vi "Autonomous Independent.vi"   [LabVIEW 2017]
doc: "This VI is called when autonomous begins, and will automatically be terminated when autonomous ends. You can carry out timed or sensor driven robot movement independently without needing to return to the caller."
uses:
  <vilib>/Rock Robotics/WPI/Utilities/WPI_GetSetVariantRefNum.vi
  <vilib>/Rock Robotics/Network Tables/NT Read String.vi
  <vilib>/Rock Robotics/Network Tables/NT Write Numeric Array.vi
  <vilib>/Rock Robotics/WPI/RobotDrive/WPI_RobotDriveArcadeDrive_Standard(NoSaturation).vi
panel:
  # "Be sure to right-click and choose Data Operations>>Make Current Value default if you want to save the array values with the VI"
types:
  T1 = typedef "WPI_JoystickDevRef.ctl" = cluster{"Device":T2}
  T2 = typedef "WPI_JoystickDeviceEnum.ctl" = enum16{"USB 0", "USB 1", "USB 2", "USB 3", "USB 4", "USB 5"}
  T3 = typedef "WPI_RobotDriveDevRef.ctl" = cluster{"DevStatus":errorcluster, "Motors[]":T4[], "Square Inputs":bool, "Max Output":dbl}
  T4 = typedef "WPI_MotorControlDeviceRef.ctl" = cluster{"DeviceStatus":errorcluster, "Type":T5, "PWM":cluster{"PWM Channel":T6, "DeadBand":T7}, "CAN":cluster{"Device Number":u8, "SetOutput VI Ref":variant, "GetOutput VI Ref":variant, "Enable VI Ref":variant, "Disable VI Ref":variant, "Data":variant}, "Invert":bool, "DIO PWM":cluster{"PWM \"Enable\" Channel":T6, "DIOChannel":T8, "PWM Rate":dbl}}
  T5 = typedef "WPI_MotorControlType.ctl" = enum16{"PWM", "CAN", "DIO PWM"}
  T6 = typedef "FPGA_DIOPWMChannel.ctl" = enum8{"PWM 0", "PWM 1", "PWM 2", "PWM 3", "PWM 4", "PWM 5", "PWM 6", "PWM 7", "PWM 8", "PWM 9", "PWM MXP 0", "PWM MXP 1", "PWM MXP 2", "PWM MXP 3", "PWM MXP 4", "PWM MXP 5", "PWM MXP 6", "PWM MXP 7", "PWM MXP 8", "PWM MXP 9", "Invalid"}
  T7 = typedef "WPI_PWMDeadband.ctl" = cluster{"Name":string, "maxPositivePwm":i32, "minPositivePwm":i32, "centerPwm":i32, "maxNegativePwm":i32, "minNegativePwm":i32, "angularRange":u16}
  T8 = typedef "FPGA_DIOChannel.ctl" = enum8{"DIO 0", "DIO 1", "DIO 2", "DIO 3", "DIO 4", "DIO 5", "DIO 6", "DIO 7", "DIO 8", "DIO 9", "DIO MXP 0", "DIO MXP 1", "DIO MXP 2", "DIO MXP 3", "DIO MXP 4", "DIO MXP 5", "DIO MXP 6", "DIO MXP 7", "DIO MXP 8", "DIO MXP 9", "DIO MXP 10", "DIO MXP 11", "DIO MXP 12", "DIO MXP 13", "DIO MXP 14", "DIO MXP 15", "SPI Port CS1", "SPI Port CS2", "SPI Port CS3", "SPI Port MISO", "SPI Port MOSI", "Invalid"}
  T9 = typedef "WPI_SwitchDevRef.ctl" = cluster{"DevStatus":errorcluster, "DIO Channel":T8, "CntIndex":T10, "Normally Closed":bool}
  T10 = typedef "FPGA_CounterCtrSystemIndex.ctl" = enum8{"Ctr 0", "Ctr 1", "Ctr 2", "Ctr 3", "Ctr 4", "Ctr 5", "Ctr 6", "Ctr 7", "Invalid"}
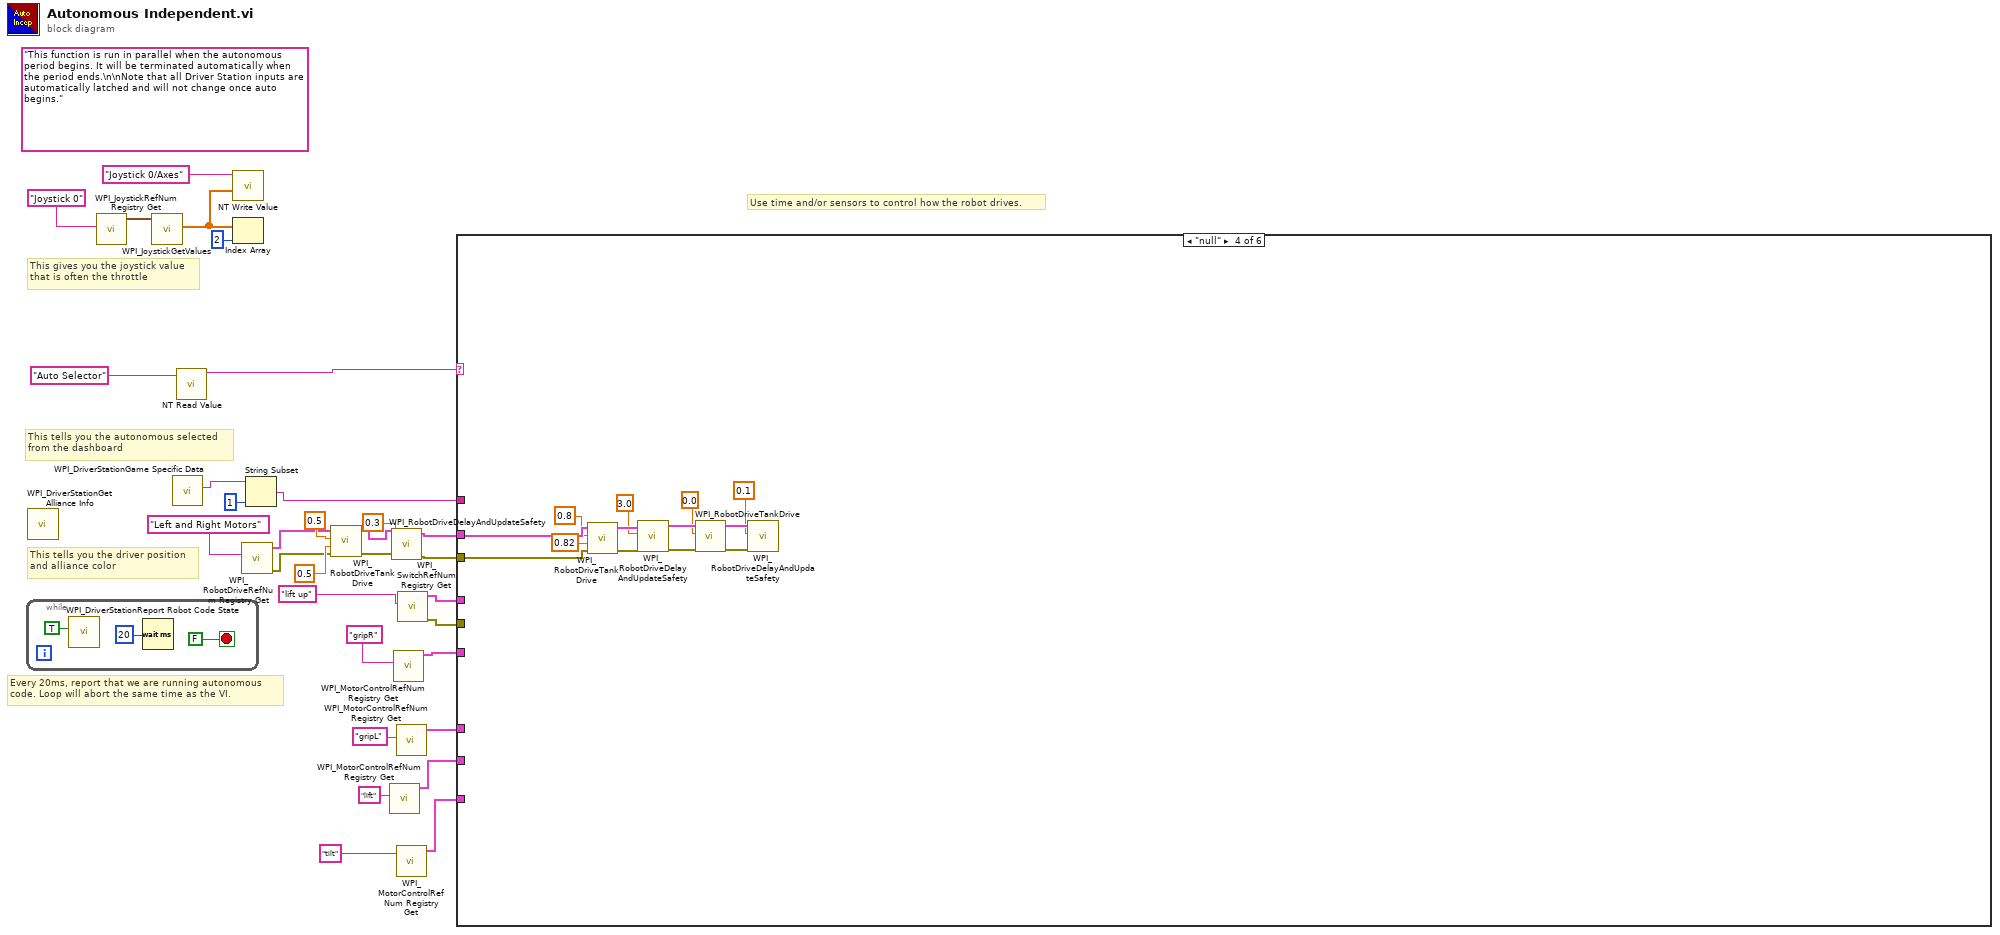
[diagram p0: block diagram]
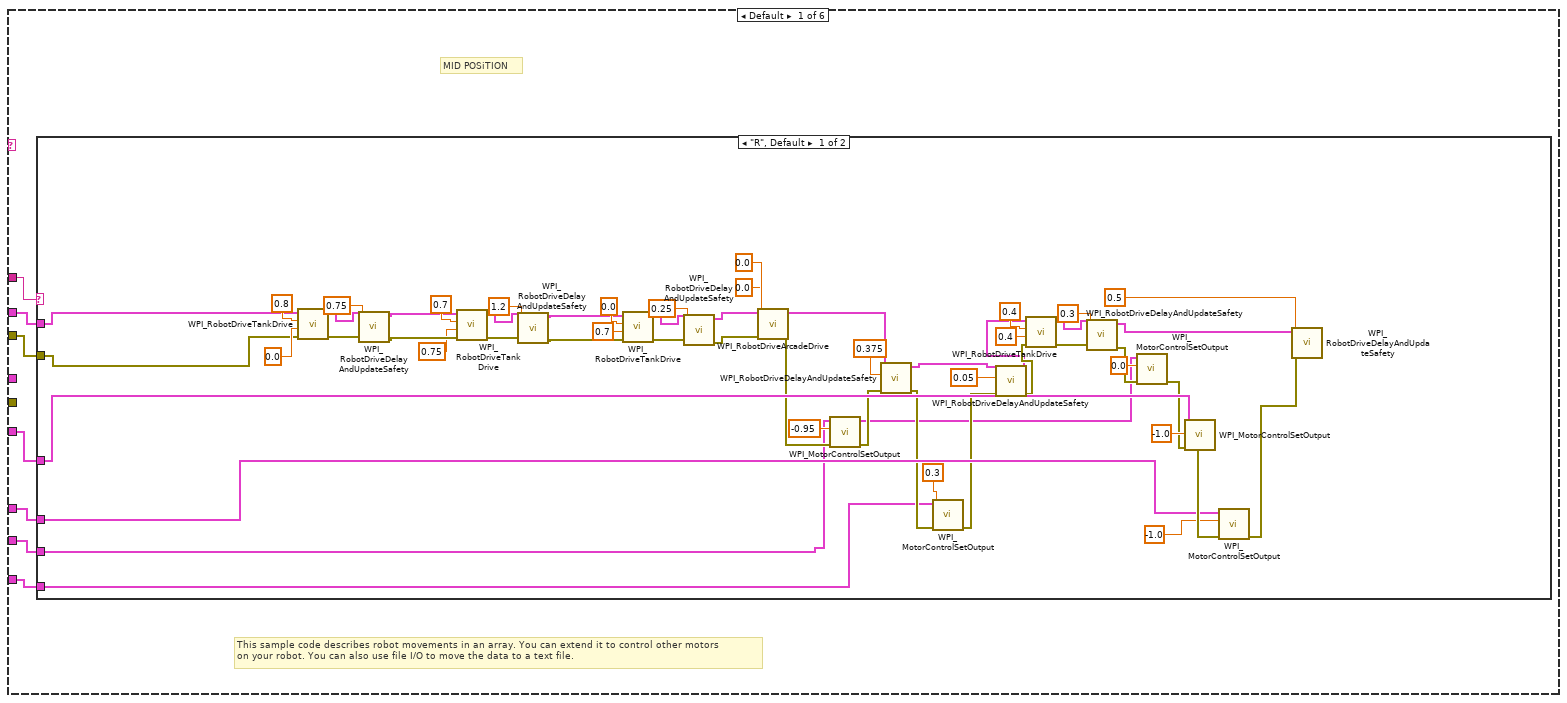
[diagram p2: hidden frame]
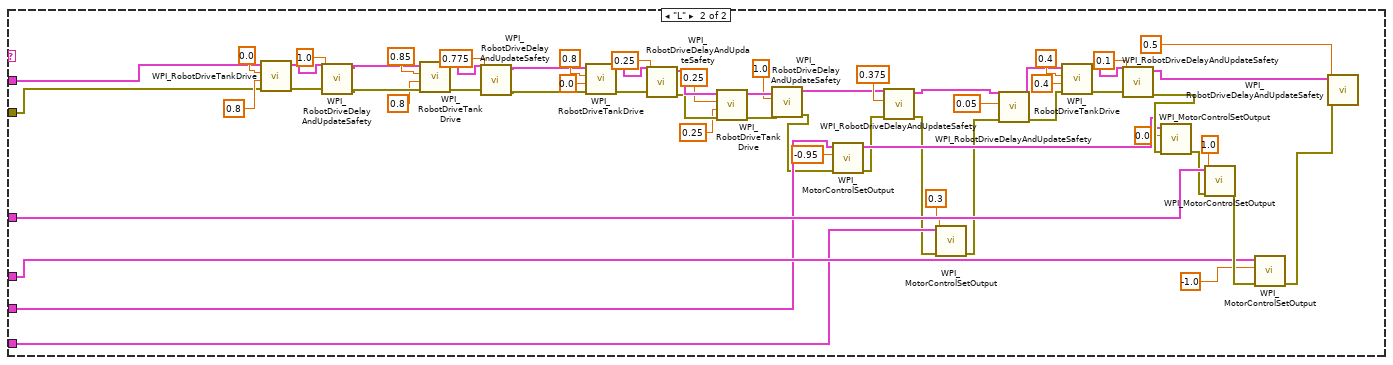
[diagram p3: hidden frame]
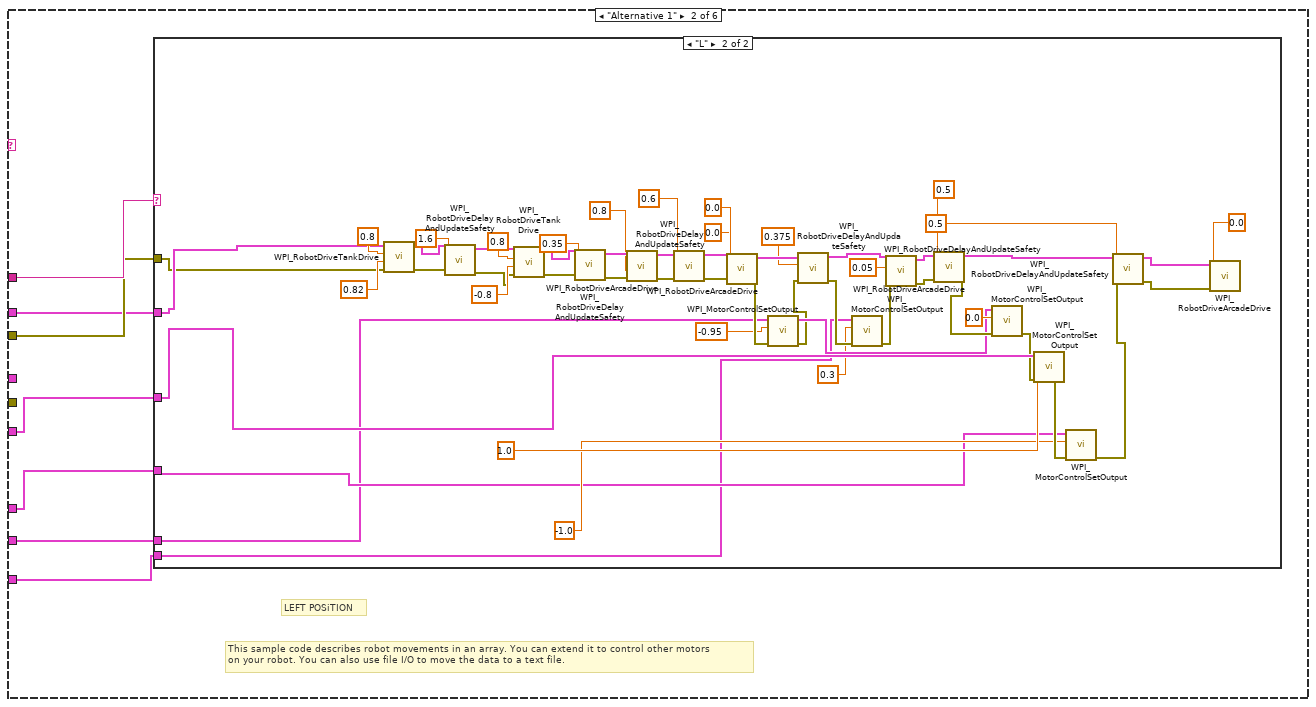
[diagram p4: hidden frame]
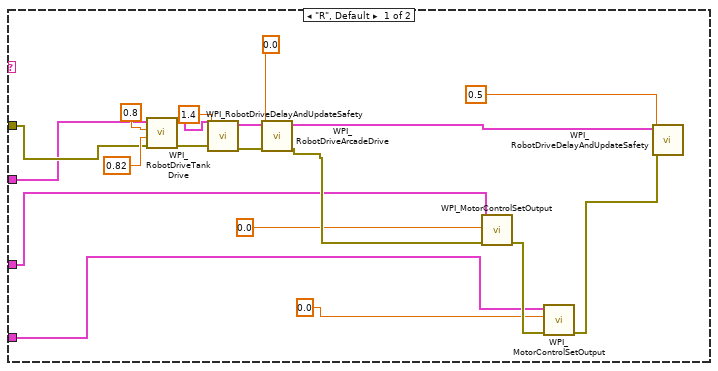
[diagram p5: hidden frame]
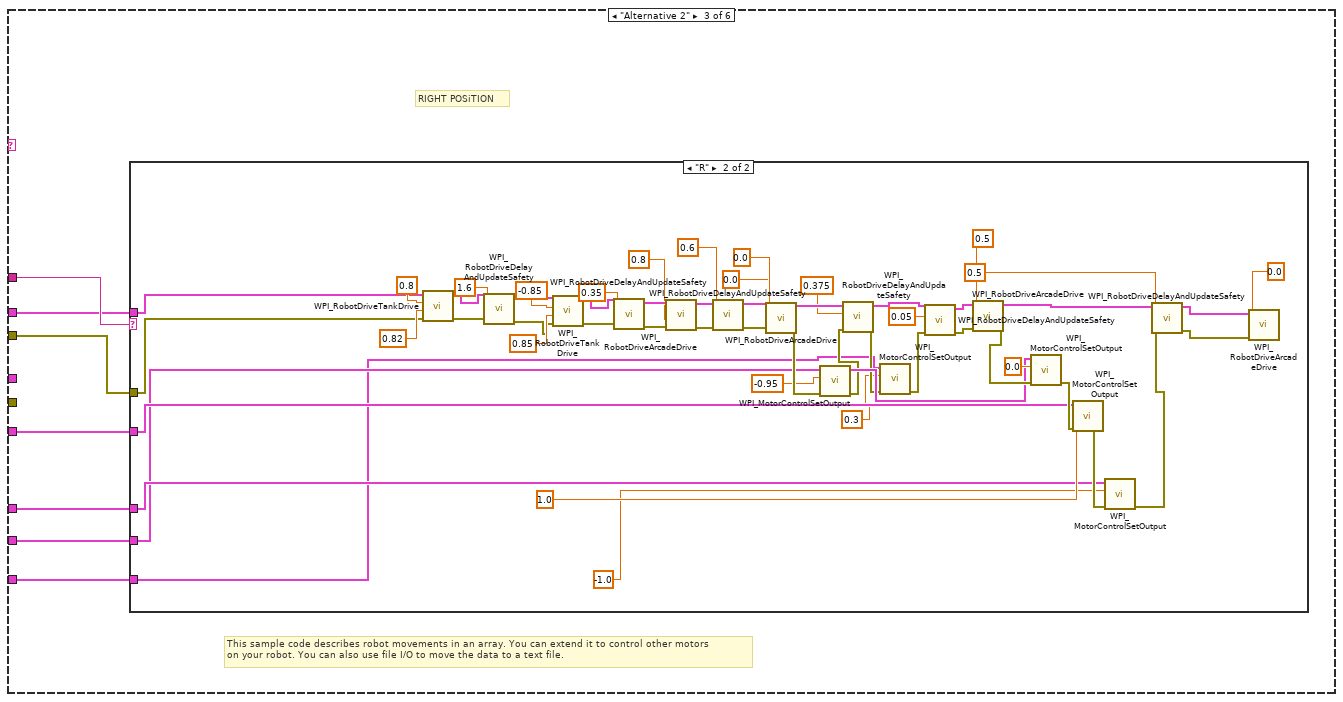
[diagram p6: hidden frame]
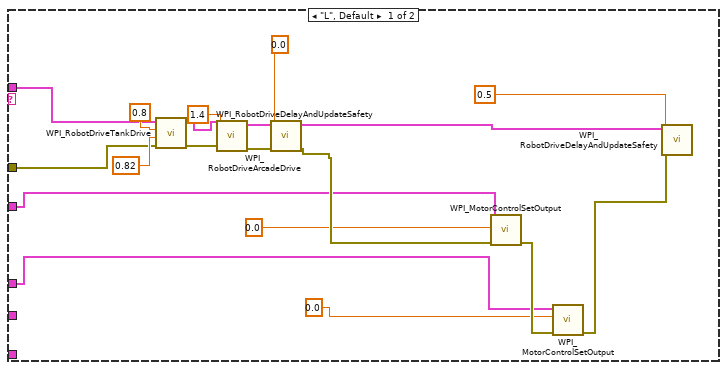
[diagram p7: hidden frame]
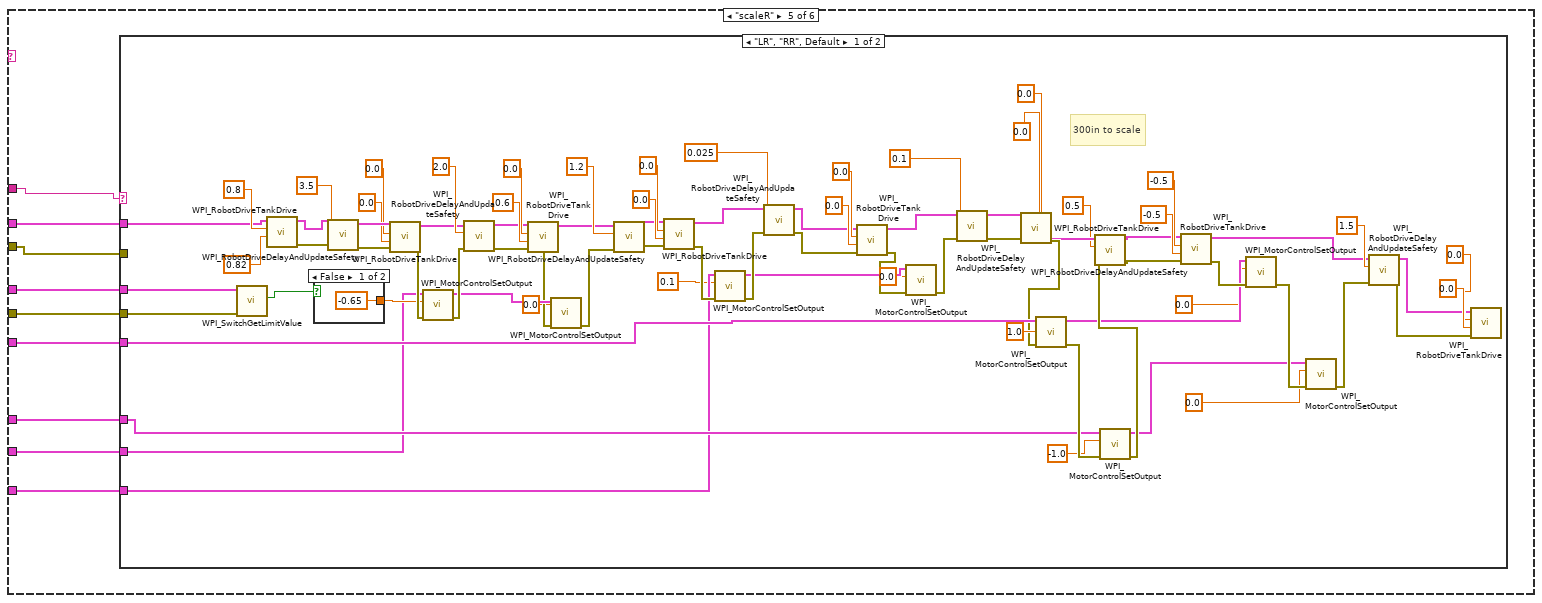
[diagram p8: hidden frame]
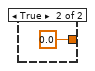
[diagram p9: hidden frame]
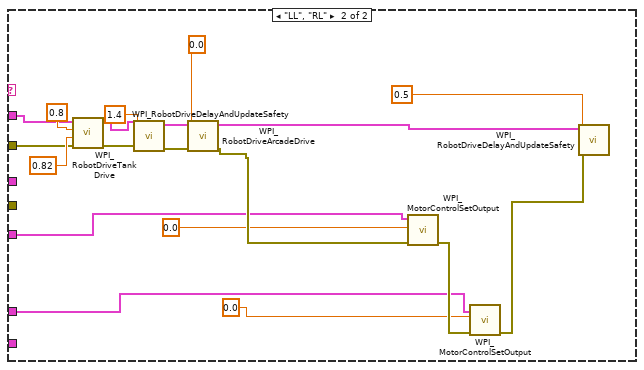
[diagram p10: hidden frame]
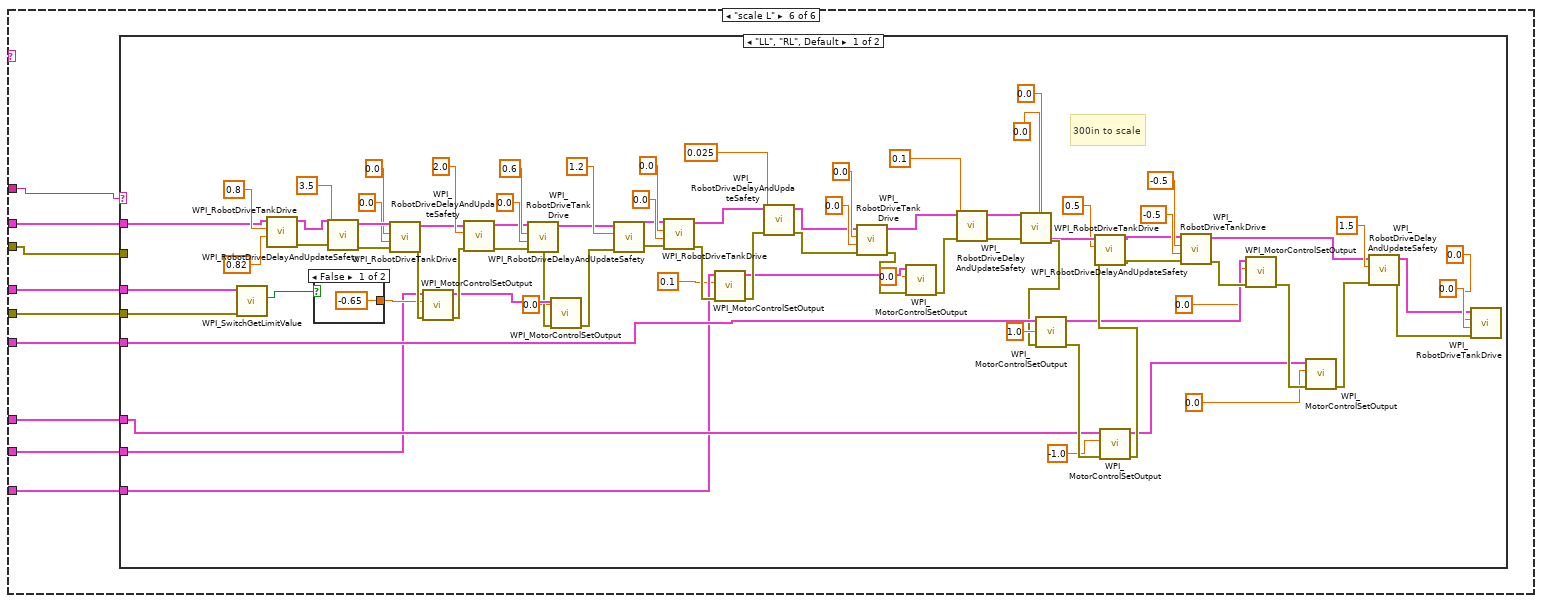
[diagram p11: hidden frame]
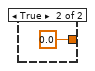
[diagram p12: hidden frame]
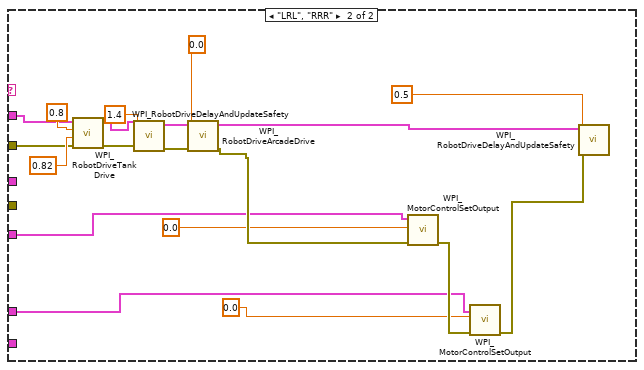
[diagram p13: hidden frame]
diagram:
  (unwired) "This function is run in parallel when the autonomous period begins. It will be terminated automatically when the period ends.\n\nNote that all Driver Station inputs are automatically latched and will not change once auto begins."
  # "This tells you the autonomous selected\nfrom the dashboard"
  # "Every 20ms, report that we are running autonomous\ncode. Loop will abort the same time as the VI."
  # "This gives you the joystick value\nthat is often the throttle"
  # "Use time and/or sensors to control how the robot drives."
  # "This tells you the driver position\nand alliance color"
  n1 = while {
    stop <- FALSE stop-if-true
    n2 = call <vilib>:"WPI_DriverStationReport Robot Code State.vi"("Autonomous"=TRUE) -> ()  [unwired: 10 in, 1 out]
    n3 = Wait (ms)(milliseconds to wait=u32 20) -> ()  [unwired: 1 out]
  }
  n4 = call <vilib>:"WPI_DriverStationGet Alliance Info.vi"() -> ()  [unwired: 12 out]
  n5 = call <vilib>:"WPI_JoystickRefNum Registry Get.vi"("refnum name"="Joystick 0") -> ("JoystickDevRef"=w30:T1)  [unwired: 1 in, 9 out]
  n6 = call <vilib>:"WPI_JoystickGetValues.vi"("JoystickDevRef"=w30) -> ("Axes"=w26:dbl[])  [unwired: 6 in, 4 out]
  n7 = call <vilib>:"WPI_DriverStationGame Specific Data.vi"() -> ("Game Specific Data"=w24:string)  [unwired: 11 in]
  n8 = call-poly <vilib>:"NT Read Value.vi"("Name"="Auto Selector") -> ("String"=w27:string)  [unwired: 9 in, 1 out]
  n9 = call-poly <vilib>:"NT Write Value.vi"("Numeric Array"=w26, "Name"="Joystick 0/Axes") -> ()  [unwired: 9 in, 1 out]
  n10 = Index Array(array=w26, index=2) -> ()  [unwired: 1 out]
  n11 = call <vilib>:"WPI_RobotDriveRefNum Registry Get.vi"("refnum name"="Left and Right Motors") -> ("error out"=w6:errorcluster, "RobotDriveDevRef"=w5:T3)  [unwired: 1 in, 8 out]
  n12 = String Subset(string=w24, length (rest)=1 ("length (rest)")) -> (substring=w22:string)  [unwired: 1 in]
  n13 = call <vilib>:"WPI_RobotDriveTankDrive.vi"("error in (no error)"=w6, "Right axis value"=0.5 ("Y axis value"), "Left axis value"=0.5 ("X axis value"), "RobotDriveDevRef"=w5) -> ("error out"=w10:errorcluster, "RobotDriveDevRef"=w9:T3)  [unwired: 5 in, 1 out]
  n14 = call <vilib>:"WPI_MotorControlRefNum Registry Get.vi"("refnum name"="lift") -> ("MotorControlDevRef"=w12:T4)  [unwired: 9 in, 1 out]
  n15 = call <vilib>:"WPI_RobotDriveDelayAndUpdateSafety.vi"("error in (no error)"=w10, "Delay (s)"=0.3, "RobotDriveDevRef"=w9) -> ("error out"=w3:errorcluster, "RobotDriveDevRef 2"=w4:T3)  [unwired: 7 in]
  n16 = call <vilib>:"WPI_MotorControlRefNum Registry Get.vi"("refnum name"="gripR") -> ("MotorControlDevRef"=w19:T4)  [unwired: 9 in, 1 out]
  n17 = call <vilib>:"WPI_MotorControlRefNum Registry Get.vi"("refnum name"="gripL") -> ("MotorControlDevRef"=w17:T4)  [unwired: 9 in, 1 out]
  n18 = call <vilib>:"WPI_MotorControlRefNum Registry Get.vi"("refnum name"="tilt") -> ("MotorControlDevRef"=w2:T4)  [unwired: 9 in, 1 out]
  n19 = call <vilib>:"WPI_SwitchRefNum Registry Get.vi"("refnum name"="lift up") -> ("error out"=w14:errorcluster, "SwitchDevRef"=w13:T9)  [unwired: 9 in]
  n20 = case shown="\"null\"" w27 {
    tunnel: w22 -> [w41 w163 w243 _ w338 w447]
    tunnel: w3 -> [w40 w162 w242 w326 w331 w440]
    tunnel: w19 -> [w39 w161 w241 _ w335 w444]
    tunnel: w17 -> [w38 w160 w240 _ w336 w445]
    tunnel: w4 -> [w37 w159 w239 w327 w337 w446]
    tunnel: w14 -> [_ _ _ _ w334 w443]
    tunnel: w13 -> [_ _ _ _ w333 w442]
    tunnel: w12 -> [w36 w158 w238 _ w332 w441]
    tunnel: w2 -> [w35 w157 w237 _ w330 w439]
    frame Default {
      # "MID POSiTION"
      # "This sample code describes robot movements in an array. You can extend it to control other motors\non your robot. You can also use file I/O to move the data to a text file."
      n21 = case shown="\"R\", Default" w41 {
        tunnel: w40 -> [w87 w126]
        tunnel: w39 -> [w86 w125]
        tunnel: w38 -> [w85 w124]
        tunnel: w37 -> [w64 w123]
        tunnel: w36 -> [w47 w116]
        tunnel: w35 -> [w46 w111]
        frame "R", Default {
          n22 = call <vilib>:"WPI_RobotDriveTankDrive.vi"("error in (no error)"=w87, "Right axis value"=0.0 ("Y axis value"), "Left axis value"=0.8 ("X axis value"), "RobotDriveDevRef"=w64) -> ("error out"=w93:errorcluster, "RobotDriveDevRef"=w92:T3)  [unwired: 5 in, 1 out]
          n23 = call <vilib>:"WPI_RobotDriveDelayAndUpdateSafety.vi"("error in (no error)"=w93, "Delay (s)"=0.75, "RobotDriveDevRef"=w92) -> ("error out"=w79:errorcluster, "RobotDriveDevRef 2"=w80:T3)  [unwired: 7 in]
          n24 = call <vilib>:"WPI_RobotDriveTankDrive.vi"("error in (no error)"=w79, "Right axis value"=0.75, "Left axis value"=0.7 ("X axis value"), "RobotDriveDevRef"=w80) -> ("error out"=w83:errorcluster, "RobotDriveDevRef"=w82:T3)  [unwired: 5 in, 1 out]
          n25 = call <vilib>:"WPI_RobotDriveDelayAndUpdateSafety.vi"("error in (no error)"=w83, "Delay (s)"=1.2, "RobotDriveDevRef"=w82) -> ("error out"=w72:errorcluster, "RobotDriveDevRef 2"=w73:T3)  [unwired: 7 in]
          n26 = call <vilib>:"WPI_RobotDriveTankDrive.vi"("error in (no error)"=w72, "Right axis value"=0.7, "Left axis value"=0.0 ("X axis value"), "RobotDriveDevRef"=w73) -> ("error out"=w76:errorcluster, "RobotDriveDevRef"=w75:T3)  [unwired: 5 in, 1 out]
          n27 = call <vilib>:"WPI_RobotDriveDelayAndUpdateSafety.vi"("error in (no error)"=w76, "Delay (s)"=0.25, "RobotDriveDevRef"=w75) -> ("error out"=w60:errorcluster, "RobotDriveDevRef 2"=w61:T3)  [unwired: 7 in]
          n28 = call-poly <vilib>:"WPI_RobotDriveArcadeDrive.vi"("error in (no error)"=w60, "Y axis value"=0.0, "X axis value"=0.0, "RobotDriveDevRef"=w61) -> ("error out"=w52:errorcluster, "RobotDriveDevRef"=w53:T3)  [unwired: 5 in, 1 out]
          n29 = call <vilib>:"WPI_MotorControlSetOutput.vi"("error in (no error)"=w52, "Output"=-0.95, "MotorControlDevRef"=w47) -> ("error out"=w51:errorcluster, "MotorControlDevRef"=w45:T4)  [unwired: 6 in, 1 out]
          n30 = call <vilib>:"WPI_RobotDriveDelayAndUpdateSafety.vi"("error in (no error)"=w51, "Delay (s)"=0.375 ("Output"), "RobotDriveDevRef"=w53) -> ("error out"=w50:errorcluster, "RobotDriveDevRef 2"=w44:T3)  [unwired: 7 in]
          n31 = call <vilib>:"WPI_MotorControlSetOutput.vi"("error in (no error)"=w50, "Output"=0.3, "MotorControlDevRef"=w46) -> ("error out"=w49:errorcluster)  [unwired: 6 in, 2 out]
          n32 = call <vilib>:"WPI_RobotDriveDelayAndUpdateSafety.vi"("error in (no error)"=w49, "Delay (s)"=0.05, "RobotDriveDevRef"=w44) -> ("error out"=w48:errorcluster, "RobotDriveDevRef 2"=w43:T3)  [unwired: 7 in]
          n33 = call <vilib>:"WPI_RobotDriveTankDrive.vi"("error in (no error)"=w48, "Right axis value"=0.4, "Left axis value"=0.4 ("X axis value"), "RobotDriveDevRef"=w43) -> ("error out"=w69:errorcluster, "RobotDriveDevRef"=w68:T3)  [unwired: 5 in, 1 out]
          n34 = call <vilib>:"WPI_RobotDriveDelayAndUpdateSafety.vi"("error in (no error)"=w69, "Delay (s)"=0.3, "RobotDriveDevRef"=w68) -> ("error out"=w59:errorcluster, "RobotDriveDevRef 2"=w65:T3)  [unwired: 7 in]
          n35 = call <vilib>:"WPI_MotorControlSetOutput.vi"("error in (no error)"=w59, "Output"=0.0, "MotorControlDevRef"=w45) -> ("error out"=w57:errorcluster)  [unwired: 6 in, 2 out]
          n36 = call <vilib>:"WPI_MotorControlSetOutput.vi"("error in (no error)"=w57, "Output"=-1.0, "MotorControlDevRef"=w86) -> ("error out"=w95:errorcluster)  [unwired: 6 in, 2 out]
          n37 = call <vilib>:"WPI_MotorControlSetOutput.vi"("error in (no error)"=w95, "Output"=-1.0, "MotorControlDevRef"=w85) -> ("error out"=w94:errorcluster)  [unwired: 6 in, 2 out]
          n38 = call <vilib>:"WPI_RobotDriveDelayAndUpdateSafety.vi"("error in (no error)"=w94, "Delay (s)"=0.5, "RobotDriveDevRef"=w65) -> ()  [unwired: 7 in, 2 out]
        }
        frame "L" {
          n39 = call <vilib>:"WPI_RobotDriveTankDrive.vi"("error in (no error)"=w126, "Right axis value"=0.8 ("Y axis value"), "Left axis value"=0.0 ("X axis value"), "RobotDriveDevRef"=w123) -> ("error out"=w152:errorcluster, "RobotDriveDevRef"=w151:T3)  [unwired: 5 in, 1 out]
          n40 = call <vilib>:"WPI_RobotDriveDelayAndUpdateSafety.vi"("error in (no error)"=w152, "Delay (s)"=1.0, "RobotDriveDevRef"=w151) -> ("error out"=w141:errorcluster, "RobotDriveDevRef 2"=w142:T3)  [unwired: 7 in]
          n41 = call <vilib>:"WPI_RobotDriveTankDrive.vi"("error in (no error)"=w141, "Right axis value"=0.8, "Left axis value"=0.85 ("X axis value"), "RobotDriveDevRef"=w142) -> ("error out"=w145:errorcluster, "RobotDriveDevRef"=w144:T3)  [unwired: 5 in, 1 out]
          n42 = call <vilib>:"WPI_RobotDriveDelayAndUpdateSafety.vi"("error in (no error)"=w145, "Delay (s)"=0.775, "RobotDriveDevRef"=w144) -> ("error out"=w134:errorcluster, "RobotDriveDevRef 2"=w135:T3)  [unwired: 7 in]
          n43 = call <vilib>:"WPI_RobotDriveTankDrive.vi"("error in (no error)"=w134, "Right axis value"=0.0, "Left axis value"=0.8 ("X axis value"), "RobotDriveDevRef"=w135) -> ("error out"=w138:errorcluster, "RobotDriveDevRef"=w137:T3)  [unwired: 5 in, 1 out]
          n44 = call <vilib>:"WPI_RobotDriveDelayAndUpdateSafety.vi"("error in (no error)"=w138, "Delay (s)"=0.25, "RobotDriveDevRef"=w137) -> ("error out"=w119:errorcluster, "RobotDriveDevRef 2"=w120:T3)  [unwired: 7 in]
          n45 = call <vilib>:"WPI_RobotDriveTankDrive.vi"("error in (no error)"=w119, "Right axis value"=0.25 ("X axis value"), "Left axis value"=0.25 ("X axis value"), "RobotDriveDevRef"=w120) -> ("error out"=w102:errorcluster, "RobotDriveDevRef"=w104:T3)  [unwired: 5 in, 1 out]
          n46 = call <vilib>:"WPI_RobotDriveDelayAndUpdateSafety.vi"("error in (no error)"=w102, "Delay (s)"=1.0 ("X axis value"), "RobotDriveDevRef"=w104) -> ("error out"=w101:errorcluster, "RobotDriveDevRef 2"=w103:T3)  [unwired: 7 in]
          n47 = call <vilib>:"WPI_MotorControlSetOutput.vi"("error in (no error)"=w101, "Output"=-0.95, "MotorControlDevRef"=w116) -> ("error out"=w109:errorcluster, "MotorControlDevRef"=w113:T4)  [unwired: 6 in, 1 out]
          n48 = call <vilib>:"WPI_RobotDriveDelayAndUpdateSafety.vi"("error in (no error)"=w109, "Delay (s)"=0.375 ("Output"), "RobotDriveDevRef"=w103) -> ("error out"=w108:errorcluster, "RobotDriveDevRef 2"=w105:T3)  [unwired: 7 in]
          n49 = call <vilib>:"WPI_MotorControlSetOutput.vi"("error in (no error)"=w108, "Output"=0.3, "MotorControlDevRef"=w111) -> ("error out"=w107:errorcluster)  [unwired: 6 in, 2 out]
          n50 = call <vilib>:"WPI_RobotDriveDelayAndUpdateSafety.vi"("error in (no error)"=w107, "Delay (s)"=0.05, "RobotDriveDevRef"=w105) -> ("error out"=w117:errorcluster, "RobotDriveDevRef 2"=w118:T3)  [unwired: 7 in]
          n51 = call <vilib>:"WPI_RobotDriveTankDrive.vi"("error in (no error)"=w117, "Right axis value"=0.4, "Left axis value"=0.4 ("X axis value"), "RobotDriveDevRef"=w118) -> ("error out"=w131:errorcluster, "RobotDriveDevRef"=w130:T3)  [unwired: 5 in, 1 out]
          n52 = call <vilib>:"WPI_RobotDriveDelayAndUpdateSafety.vi"("error in (no error)"=w131, "Delay (s)"=0.1, "RobotDriveDevRef"=w130) -> ("error out"=w115:errorcluster, "RobotDriveDevRef 2"=w127:T3)  [unwired: 7 in]
          n53 = call <vilib>:"WPI_MotorControlSetOutput.vi"("error in (no error)"=w115, "Output"=0.0, "MotorControlDevRef"=w113) -> ("error out"=w114:errorcluster)  [unwired: 6 in, 2 out]
          n54 = call <vilib>:"WPI_MotorControlSetOutput.vi"("error in (no error)"=w114, "Output"=1.0, "MotorControlDevRef"=w125) -> ("error out"=w154:errorcluster)  [unwired: 6 in, 2 out]
          n55 = call <vilib>:"WPI_MotorControlSetOutput.vi"("error in (no error)"=w154, "Output"=-1.0, "MotorControlDevRef"=w124) -> ("error out"=w153:errorcluster)  [unwired: 6 in, 2 out]
          n56 = call <vilib>:"WPI_RobotDriveDelayAndUpdateSafety.vi"("error in (no error)"=w153, "Delay (s)"=0.5, "RobotDriveDevRef"=w127) -> ()  [unwired: 7 in, 2 out]
        }
      }
    }
    frame "Alternative 1" {
      # "LEFT POSiTION"
      # "This sample code describes robot movements in an array. You can extend it to control other motors\non your robot. You can also use file I/O to move the data to a text file."
      n57 = case shown="\"L\"" w163 {
        tunnel: w162 -> [w167 w216]
        tunnel: w161 -> [w166 w215]
        tunnel: w160 -> [w165 w214]
        tunnel: w159 -> [w164 w217]
        tunnel: w158 -> [_ w194]
        tunnel: w157 -> [_ w184]
        frame "R", Default {
          n58 = call <vilib>:"WPI_RobotDriveTankDrive.vi"("error in (no error)"=w167, "Right axis value"=0.82 ("Y axis value"), "Left axis value"=0.8 ("X axis value"), "RobotDriveDevRef"=w164) -> ("error out"=w173:errorcluster, "RobotDriveDevRef"=w172:T3)  [unwired: 5 in, 1 out]
          n59 = call <vilib>:"WPI_RobotDriveDelayAndUpdateSafety.vi"("error in (no error)"=w173, "Delay (s)"=1.4, "RobotDriveDevRef"=w172) -> ("error out"=w181:errorcluster, "RobotDriveDevRef 2"=w180:T3)  [unwired: 7 in]
          n60 = call-poly <vilib>:"WPI_RobotDriveArcadeDrive.vi"("error in (no error)"=w181, "Y axis value"=0.0, "RobotDriveDevRef"=w180) -> ("error out"=w175:errorcluster, "RobotDriveDevRef"=w178:T3)  [unwired: 6 in, 1 out]
          n61 = call <vilib>:"WPI_MotorControlSetOutput.vi"("error in (no error)"=w175, "Output"=0.0, "MotorControlDevRef"=w166) -> ("error out"=w176:errorcluster)  [unwired: 6 in, 2 out]
          n62 = call <vilib>:"WPI_MotorControlSetOutput.vi"("error in (no error)"=w176, "Output"=0.0, "MotorControlDevRef"=w165) -> ("error out"=w174:errorcluster)  [unwired: 6 in, 2 out]
          n63 = call <vilib>:"WPI_RobotDriveDelayAndUpdateSafety.vi"("error in (no error)"=w174, "Delay (s)"=0.5, "RobotDriveDevRef"=w178) -> ()  [unwired: 7 in, 2 out]
        }
        frame "L" {
          n64 = call <vilib>:"WPI_RobotDriveTankDrive.vi"("error in (no error)"=w216, "Right axis value"=0.82 ("Y axis value"), "Left axis value"=0.8 ("X axis value"), "RobotDriveDevRef"=w217) -> ("error out"=w230:errorcluster, "RobotDriveDevRef"=w229:T3)  [unwired: 5 in, 1 out]
          n65 = call <vilib>:"WPI_RobotDriveDelayAndUpdateSafety.vi"("error in (no error)"=w230, "Delay (s)"=1.6, "RobotDriveDevRef"=w229) -> ("error out"=w218:errorcluster, "RobotDriveDevRef 2"=w219:T3)  [unwired: 7 in]
          n66 = call <vilib>:"WPI_RobotDriveTankDrive.vi"("error in (no error)"=w218, "Right axis value"=-0.8 ("Y axis value"), "Left axis value"=0.8 ("X axis value"), "RobotDriveDevRef"=w219) -> ("error out"=w223:errorcluster, "RobotDriveDevRef"=w222:T3)  [unwired: 5 in, 1 out]
          n67 = call <vilib>:"WPI_RobotDriveDelayAndUpdateSafety.vi"("error in (no error)"=w223, "Delay (s)"=0.35, "RobotDriveDevRef"=w222) -> ("error out"=w209:errorcluster, "RobotDriveDevRef 2"=w210:T3)  [unwired: 7 in]
          n68 = call-poly <vilib>:"WPI_RobotDriveArcadeDrive.vi"("error in (no error)"=w209, "Y axis value"=0.8, "RobotDriveDevRef"=w210) -> ("error out"=w206:errorcluster, "RobotDriveDevRef"=w207:T3)  [unwired: 6 in, 1 out]
          n69 = call <vilib>:"WPI_RobotDriveDelayAndUpdateSafety.vi"("error in (no error)"=w206, "Delay (s)"=0.6, "RobotDriveDevRef"=w207) -> ("error out"=w204:errorcluster, "RobotDriveDevRef 2"=w203:T3)  [unwired: 7 in]
          n70 = call-poly <vilib>:"WPI_RobotDriveArcadeDrive.vi"("error in (no error)"=w204, "Y axis value"=0.0, "X axis value"=0.0, "RobotDriveDevRef"=w203) -> ("error out"=w195:errorcluster, "RobotDriveDevRef"=w191:T3)  [unwired: 5 in, 1 out]
          n71 = call <vilib>:"WPI_MotorControlSetOutput.vi"("error in (no error)"=w195, "Output"=-0.95 ("Delay (s)"), "MotorControlDevRef"=w194) -> ("error out"=w190:errorcluster, "MotorControlDevRef"=w193:T4)  [unwired: 6 in, 1 out]
          n72 = call <vilib>:"WPI_RobotDriveDelayAndUpdateSafety.vi"("error in (no error)"=w190, "Delay (s)"=0.375, "RobotDriveDevRef"=w191) -> ("error out"=w187:errorcluster, "RobotDriveDevRef 2"=w188:T3)  [unwired: 7 in]
          n73 = call <vilib>:"WPI_MotorControlSetOutput.vi"("error in (no error)"=w187, "Output"=0.3 ("Delay (s)"), "MotorControlDevRef"=w184) -> ("error out"=w186:errorcluster)  [unwired: 6 in, 2 out]
          n74 = call <vilib>:"WPI_RobotDriveDelayAndUpdateSafety.vi"("error in (no error)"=w186, "Delay (s)"=0.05, "RobotDriveDevRef"=w188) -> ("error out"=w183:errorcluster, "RobotDriveDevRef 2"=w202:T3)  [unwired: 7 in]
          n75 = call-poly <vilib>:"WPI_RobotDriveArcadeDrive.vi"("error in (no error)"=w183, "Y axis value"=0.5, "RobotDriveDevRef"=w202) -> ("error out"=w197:errorcluster, "RobotDriveDevRef"=w234:T3)  [unwired: 6 in, 1 out]
          n76 = call <vilib>:"WPI_MotorControlSetOutput.vi"("error in (no error)"=w197, "Output"=0.0, "MotorControlDevRef"=w193) -> ("error out"=w196:errorcluster)  [unwired: 6 in, 2 out]
          n77 = call <vilib>:"WPI_MotorControlSetOutput.vi"("error in (no error)"=w196, "Output"=1.0, "MotorControlDevRef"=w215) -> ("error out"=w232:errorcluster)  [unwired: 6 in, 2 out]
          n78 = call <vilib>:"WPI_MotorControlSetOutput.vi"("error in (no error)"=w232, "Output"=-1.0, "MotorControlDevRef"=w214) -> ("error out"=w231:errorcluster)  [unwired: 6 in, 2 out]
          n79 = call <vilib>:"WPI_RobotDriveDelayAndUpdateSafety.vi"("error in (no error)"=w231, "Delay (s)"=0.5, "RobotDriveDevRef"=w234) -> ("error out"=w211:errorcluster, "RobotDriveDevRef 2"=w212:T3)  [unwired: 7 in]
          n80 = call-poly <vilib>:"WPI_RobotDriveArcadeDrive.vi"("error in (no error)"=w211, "Y axis value"=0.0, "RobotDriveDevRef"=w212) -> ()  [unwired: 6 in, 3 out]
        }
      }
    }
    frame "Alternative 2" {
      # "RIGHT POSiTION"
      # "This sample code describes robot movements in an array. You can extend it to control other motors\non your robot. You can also use file I/O to move the data to a text file."
      n81 = case shown="\"R\"" w243 {
        tunnel: w242 -> [w245 w278]
        tunnel: w241 -> [w246 w277]
        tunnel: w240 -> [w247 w276]
        tunnel: w239 -> [w244 w279]
        tunnel: w238 -> [_ w274]
        tunnel: w237 -> [_ w263]
        frame "L", Default {
          n82 = call <vilib>:"WPI_RobotDriveTankDrive.vi"("error in (no error)"=w245, "Right axis value"=0.82 ("Y axis value"), "Left axis value"=0.8 ("X axis value"), "RobotDriveDevRef"=w244) -> ("error out"=w253:errorcluster, "RobotDriveDevRef"=w252:T3)  [unwired: 5 in, 1 out]
          n83 = call <vilib>:"WPI_RobotDriveDelayAndUpdateSafety.vi"("error in (no error)"=w253, "Delay (s)"=1.4, "RobotDriveDevRef"=w252) -> ("error out"=w261:errorcluster, "RobotDriveDevRef 2"=w260:T3)  [unwired: 7 in]
          n84 = call-poly <vilib>:"WPI_RobotDriveArcadeDrive.vi"("error in (no error)"=w261, "Y axis value"=0.0, "RobotDriveDevRef"=w260) -> ("error out"=w255:errorcluster, "RobotDriveDevRef"=w258:T3)  [unwired: 6 in, 1 out]
          n85 = call <vilib>:"WPI_MotorControlSetOutput.vi"("error in (no error)"=w255, "Output"=0.0, "MotorControlDevRef"=w246) -> ("error out"=w256:errorcluster)  [unwired: 6 in, 2 out]
          n86 = call <vilib>:"WPI_MotorControlSetOutput.vi"("error in (no error)"=w256, "Output"=0.0, "MotorControlDevRef"=w247) -> ("error out"=w254:errorcluster)  [unwired: 6 in, 2 out]
          n87 = call <vilib>:"WPI_RobotDriveDelayAndUpdateSafety.vi"("error in (no error)"=w254, "Delay (s)"=0.5, "RobotDriveDevRef"=w258) -> ()  [unwired: 7 in, 2 out]
        }
        frame "R" {
          n88 = call <vilib>:"WPI_RobotDriveTankDrive.vi"("error in (no error)"=w278, "Right axis value"=0.82 ("Y axis value"), "Left axis value"=0.8 ("X axis value"), "RobotDriveDevRef"=w279) -> ("error out"=w310:errorcluster, "RobotDriveDevRef"=w309:T3)  [unwired: 5 in, 1 out]
          n89 = call <vilib>:"WPI_RobotDriveDelayAndUpdateSafety.vi"("error in (no error)"=w310, "Delay (s)"=1.6, "RobotDriveDevRef"=w309) -> ("error out"=w298:errorcluster, "RobotDriveDevRef 2"=w299:T3)  [unwired: 7 in]
          n90 = call <vilib>:"WPI_RobotDriveTankDrive.vi"("error in (no error)"=w298, "Right axis value"=0.85 ("Y axis value"), "Left axis value"=-0.85 ("X axis value"), "RobotDriveDevRef"=w299) -> ("error out"=w303:errorcluster, "RobotDriveDevRef"=w302:T3)  [unwired: 5 in, 1 out]
          n91 = call <vilib>:"WPI_RobotDriveDelayAndUpdateSafety.vi"("error in (no error)"=w303, "Delay (s)"=0.35, "RobotDriveDevRef"=w302) -> ("error out"=w293:errorcluster, "RobotDriveDevRef 2"=w294:T3)  [unwired: 7 in]
          n92 = call-poly <vilib>:"WPI_RobotDriveArcadeDrive.vi"("error in (no error)"=w293, "Y axis value"=0.8, "RobotDriveDevRef"=w294) -> ("error out"=w290:errorcluster, "RobotDriveDevRef"=w291:T3)  [unwired: 6 in, 1 out]
          n93 = call <vilib>:"WPI_RobotDriveDelayAndUpdateSafety.vi"("error in (no error)"=w290, "Delay (s)"=0.6, "RobotDriveDevRef"=w291) -> ("error out"=w288:errorcluster, "RobotDriveDevRef 2"=w287:T3)  [unwired: 7 in]
          n94 = call-poly <vilib>:"WPI_RobotDriveArcadeDrive.vi"("error in (no error)"=w288, "Y axis value"=0.0, "X axis value"=0.0, "RobotDriveDevRef"=w287) -> ("error out"=w275:errorcluster, "RobotDriveDevRef"=w269:T3)  [unwired: 5 in, 1 out]
          n95 = call <vilib>:"WPI_MotorControlSetOutput.vi"("error in (no error)"=w275, "Output"=-0.95 ("Delay (s)"), "MotorControlDevRef"=w274) -> ("error out"=w272:errorcluster, "MotorControlDevRef"=w273:T4)  [unwired: 6 in, 1 out]
          n96 = call <vilib>:"WPI_RobotDriveDelayAndUpdateSafety.vi"("error in (no error)"=w272, "Delay (s)"=0.375, "RobotDriveDevRef"=w269) -> ("error out"=w271:errorcluster, "RobotDriveDevRef 2"=w268:T3)  [unwired: 7 in]
          n97 = call <vilib>:"WPI_MotorControlSetOutput.vi"("error in (no error)"=w271, "Output"=0.3 ("Delay (s)"), "MotorControlDevRef"=w263) -> ("error out"=w270:errorcluster)  [unwired: 6 in, 2 out]
          n98 = call <vilib>:"WPI_RobotDriveDelayAndUpdateSafety.vi"("error in (no error)"=w270, "Delay (s)"=0.05, "RobotDriveDevRef"=w268) -> ("error out"=w264:errorcluster, "RobotDriveDevRef 2"=w286:T3)  [unwired: 7 in]
          n99 = call-poly <vilib>:"WPI_RobotDriveArcadeDrive.vi"("error in (no error)"=w264, "Y axis value"=0.5, "RobotDriveDevRef"=w286) -> ("error out"=w281:errorcluster, "RobotDriveDevRef"=w314:T3)  [unwired: 6 in, 1 out]
          n100 = call <vilib>:"WPI_MotorControlSetOutput.vi"("error in (no error)"=w281, "Output"=0.0, "MotorControlDevRef"=w273) -> ("error out"=w280:errorcluster)  [unwired: 6 in, 2 out]
          n101 = call <vilib>:"WPI_MotorControlSetOutput.vi"("error in (no error)"=w280, "Output"=1.0, "MotorControlDevRef"=w277) -> ("error out"=w312:errorcluster)  [unwired: 6 in, 2 out]
          n102 = call <vilib>:"WPI_MotorControlSetOutput.vi"("error in (no error)"=w312, "Output"=-1.0, "MotorControlDevRef"=w276) -> ("error out"=w311:errorcluster)  [unwired: 6 in, 2 out]
          n103 = call <vilib>:"WPI_RobotDriveDelayAndUpdateSafety.vi"("error in (no error)"=w311, "Delay (s)"=0.5, "RobotDriveDevRef"=w314) -> ("error out"=w295:errorcluster, "RobotDriveDevRef 2"=w296:T3)  [unwired: 7 in]
          n104 = call-poly <vilib>:"WPI_RobotDriveArcadeDrive.vi"("error in (no error)"=w295, "Y axis value"=0.0, "RobotDriveDevRef"=w296) -> ()  [unwired: 6 in, 3 out]
        }
      }
    }
    frame "null" {
      n105 = call <vilib>:"WPI_RobotDriveTankDrive.vi"("error in (no error)"=w326, "Right axis value"=0.82, "Left axis value"=0.8 ("Output"), "RobotDriveDevRef"=w327) -> ("error out"=w329:errorcluster, "RobotDriveDevRef"=w328:T3)  [unwired: 5 in, 1 out]
      n106 = call <vilib>:"WPI_RobotDriveDelayAndUpdateSafety.vi"("error in (no error)"=w329, "Delay (s)"=3.0 ("Output"), "RobotDriveDevRef"=w328) -> ("error out"=w325:errorcluster, "RobotDriveDevRef 2"=w324:T3)  [unwired: 7 in]
      n107 = call <vilib>:"WPI_RobotDriveTankDrive.vi"("error in (no error)"=w325, "Left axis value"=0.0 ("Output"), "RobotDriveDevRef"=w324) -> ("error out"=w323:errorcluster, "RobotDriveDevRef"=w322:T3)  [unwired: 6 in, 1 out]
      n108 = call <vilib>:"WPI_RobotDriveDelayAndUpdateSafety.vi"("error in (no error)"=w323, "Delay (s)"=0.1 ("Output"), "RobotDriveDevRef"=w322) -> ()  [unwired: 7 in, 2 out]
    }
    frame "scaleR" {
      n109 = case shown="\"LR\", \"RR\", Default" w338 {
        tunnel: w337 -> [w408 w422]
        tunnel: w336 -> [w388 w420]
        tunnel: w335 -> [w389 w421]
        tunnel: w334 -> [w385 _]
        tunnel: w333 -> [w384 _]
        tunnel: w332 -> [w383 _]
        tunnel: w331 -> [_ w423]
        tunnel: w330 -> [w352 _]
        frame "LR", "RR", Default {
          # "300in to scale"
          n110 = call <vilib>:"WPI_SwitchGetLimitValue.vi"("error in (no error)"=w385, "SwitchDevRef"=w384) -> ("Switch Pressed"=w386:bool)  [unwired: 7 in, 2 out]
          n111 = call <vilib>:"WPI_RobotDriveTankDrive.vi"("Right axis value"=0.82 ("Y axis value"), "Left axis value"=0.8 ("X axis value"), "RobotDriveDevRef"=w408) -> ("error out"=w414:errorcluster, "RobotDriveDevRef"=w413:T3)  [unwired: 6 in, 1 out]
          n112 = case shown="False" w386 {
            tunnel: [-0.65 ("Output") 0.0 ("Output")] -> w387
            frame False {
            }
            frame True {
            }
          }
          n113 = call <vilib>:"WPI_RobotDriveDelayAndUpdateSafety.vi"("error in (no error)"=w414, "Delay (s)"=3.5, "RobotDriveDevRef"=w413) -> ("error out"=w406:errorcluster, "RobotDriveDevRef 2"=w407:T3)  [unwired: 7 in]
          n114 = call <vilib>:"WPI_RobotDriveTankDrive.vi"("error in (no error)"=w406, "Right axis value"=0.0, "Left axis value"=0.0, "RobotDriveDevRef"=w407) -> ("error out"=w403:errorcluster, "RobotDriveDevRef"=w401:T3)  [unwired: 5 in, 1 out]
          n115 = call <vilib>:"WPI_MotorControlSetOutput.vi"("error in (no error)"=w403, "Output"=w387, "MotorControlDevRef"=w383) -> ("error out"=w400:errorcluster, "MotorControlDevRef"=w382:T4)  [unwired: 6 in, 1 out]
          n116 = call <vilib>:"WPI_RobotDriveDelayAndUpdateSafety.vi"("error in (no error)"=w400, "Delay (s)"=2.0, "RobotDriveDevRef"=w401) -> ("error out"=w394:errorcluster, "RobotDriveDevRef 2"=w395:T3)  [unwired: 7 in]
          n117 = call <vilib>:"WPI_RobotDriveTankDrive.vi"("error in (no error)"=w394, "Right axis value"=0.6, "Left axis value"=0.0, "RobotDriveDevRef"=w395) -> ("error out"=w381:errorcluster, "RobotDriveDevRef"=w396:T3)  [unwired: 5 in, 1 out]
          n118 = call <vilib>:"WPI_MotorControlSetOutput.vi"("error in (no error)"=w381, "Output"=0.0, "MotorControlDevRef"=w382) -> ("error out"=w355:errorcluster)  [unwired: 6 in, 2 out]
          n119 = call <vilib>:"WPI_RobotDriveDelayAndUpdateSafety.vi"("error in (no error)"=w355, "Delay (s)"=1.2, "RobotDriveDevRef"=w396) -> ("error out"=w390:errorcluster, "RobotDriveDevRef 2"=w391:T3)  [unwired: 7 in]
          n120 = call <vilib>:"WPI_RobotDriveTankDrive.vi"("error in (no error)"=w390, "Right axis value"=0.0, "Left axis value"=0.0, "RobotDriveDevRef"=w391) -> ("error out"=w354:errorcluster, "RobotDriveDevRef"=w366:T3)  [unwired: 5 in, 1 out]
          n121 = call <vilib>:"WPI_MotorControlSetOutput.vi"("error in (no error)"=w354, "Output"=0.1, "MotorControlDevRef"=w352) -> ("error out"=w353:errorcluster, "MotorControlDevRef"=w344:T4)  [unwired: 6 in, 1 out]
          n122 = call <vilib>:"WPI_RobotDriveDelayAndUpdateSafety.vi"("error in (no error)"=w353, "Delay (s)"=0.025, "RobotDriveDevRef"=w366) -> ("error out"=w345:errorcluster, "RobotDriveDevRef 2"=w346:T3)  [unwired: 7 in]
          n123 = call <vilib>:"WPI_RobotDriveTankDrive.vi"("error in (no error)"=w345, "Right axis value"=0.0, "Left axis value"=0.0, "RobotDriveDevRef"=w346) -> ("error out"=w342:errorcluster, "RobotDriveDevRef"=w349:T3)  [unwired: 5 in, 1 out]
          n124 = call <vilib>:"WPI_MotorControlSetOutput.vi"("error in (no error)"=w342, "Output"=0.0, "MotorControlDevRef"=w344) -> ("error out"=w341:errorcluster)  [unwired: 6 in, 2 out]
          n125 = call <vilib>:"WPI_RobotDriveDelayAndUpdateSafety.vi"("error in (no error)"=w341, "Delay (s)"=0.1, "RobotDriveDevRef"=w349) -> ("error out"=w339:errorcluster, "RobotDriveDevRef 2"=w340:T3)  [unwired: 7 in]
          n126 = call <vilib>:"WPI_RobotDriveTankDrive.vi"("error in (no error)"=w339, "Right axis value"=0.0, "Left axis value"=0.0, "RobotDriveDevRef"=w340) -> ("error out"=w365:errorcluster, "RobotDriveDevRef"=w364:T3)  [unwired: 5 in, 1 out]
          n127 = call <vilib>:"WPI_MotorControlSetOutput.vi"("error in (no error)"=w365, "Output"=1.0, "MotorControlDevRef"=w389) -> ("error out"=w416:errorcluster, "MotorControlDevRef"=w373:T4)  [unwired: 6 in, 1 out]
          n128 = call <vilib>:"WPI_MotorControlSetOutput.vi"("error in (no error)"=w416, "Output"=-1.0, "MotorControlDevRef"=w388) -> ("error out"=w415:errorcluster, "MotorControlDevRef"=w372:T4)  [unwired: 6 in, 1 out]
          n129 = call <vilib>:"WPI_RobotDriveDelayAndUpdateSafety.vi"("error in (no error)"=w415, "Delay (s)"=0.5, "RobotDriveDevRef"=w364) -> ("error out"=w376:errorcluster, "RobotDriveDevRef 2"=w377:T3)  [unwired: 7 in]
          n130 = call <vilib>:"WPI_RobotDriveTankDrive.vi"("error in (no error)"=w376, "Right axis value"=-0.5, "Left axis value"=-0.5, "RobotDriveDevRef"=w377) -> ("error out"=w374:errorcluster, "RobotDriveDevRef"=w361:T3)  [unwired: 5 in, 1 out]
          n131 = call <vilib>:"WPI_MotorControlSetOutput.vi"("error in (no error)"=w374, "Output"=0.0, "MotorControlDevRef"=w373) -> ("error out"=w375:errorcluster)  [unwired: 6 in, 2 out]
          n132 = call <vilib>:"WPI_MotorControlSetOutput.vi"("error in (no error)"=w375, "Output"=0.0, "MotorControlDevRef"=w372) -> ("error out"=w360:errorcluster)  [unwired: 6 in, 2 out]
          n133 = call <vilib>:"WPI_RobotDriveDelayAndUpdateSafety.vi"("error in (no error)"=w360, "Delay (s)"=1.5, "RobotDriveDevRef"=w361) -> ("error out"=w356:errorcluster, "RobotDriveDevRef 2"=w357:T3)  [unwired: 7 in]
          n134 = call <vilib>:"WPI_RobotDriveTankDrive.vi"("error in (no error)"=w356, "Right axis value"=0.0, "Left axis value"=0.0, "RobotDriveDevRef"=w357) -> ()  [unwired: 5 in, 3 out]
        }
        frame "LL", "RL" {
          n135 = call <vilib>:"WPI_RobotDriveTankDrive.vi"("error in (no error)"=w423, "Right axis value"=0.82 ("Y axis value"), "Left axis value"=0.8 ("X axis value"), "RobotDriveDevRef"=w422) -> ("error out"=w429:errorcluster, "RobotDriveDevRef"=w428:T3)  [unwired: 5 in, 1 out]
          n136 = call <vilib>:"WPI_RobotDriveDelayAndUpdateSafety.vi"("error in (no error)"=w429, "Delay (s)"=1.4, "RobotDriveDevRef"=w428) -> ("error out"=w437:errorcluster, "RobotDriveDevRef 2"=w436:T3)  [unwired: 7 in]
          n137 = call-poly <vilib>:"WPI_RobotDriveArcadeDrive.vi"("error in (no error)"=w437, "Y axis value"=0.0, "RobotDriveDevRef"=w436) -> ("error out"=w431:errorcluster, "RobotDriveDevRef"=w434:T3)  [unwired: 6 in, 1 out]
          n138 = call <vilib>:"WPI_MotorControlSetOutput.vi"("error in (no error)"=w431, "Output"=0.0, "MotorControlDevRef"=w421) -> ("error out"=w432:errorcluster)  [unwired: 6 in, 2 out]
          n139 = call <vilib>:"WPI_MotorControlSetOutput.vi"("error in (no error)"=w432, "Output"=0.0, "MotorControlDevRef"=w420) -> ("error out"=w430:errorcluster)  [unwired: 6 in, 2 out]
          n140 = call <vilib>:"WPI_RobotDriveDelayAndUpdateSafety.vi"("error in (no error)"=w430, "Delay (s)"=0.5, "RobotDriveDevRef"=w434) -> ()  [unwired: 7 in, 2 out]
        }
      }
    }
    frame "scale L" {
      n141 = case shown="\"LL\", \"RL\", Default" w447 {
        tunnel: w446 -> [w517 w531]
        tunnel: w445 -> [w497 w529]
        tunnel: w444 -> [w498 w530]
        tunnel: w443 -> [w494 _]
        tunnel: w442 -> [w493 _]
        tunnel: w441 -> [w492 _]
        tunnel: w440 -> [_ w532]
        tunnel: w439 -> [w461 _]
        frame "LL", "RL", Default {
          # "300in to scale"
          n142 = call <vilib>:"WPI_SwitchGetLimitValue.vi"("error in (no error)"=w494, "SwitchDevRef"=w493) -> ("Switch Pressed"=w495:bool)  [unwired: 7 in, 2 out]
          n143 = call <vilib>:"WPI_RobotDriveTankDrive.vi"("Right axis value"=0.82 ("Y axis value"), "Left axis value"=0.8 ("X axis value"), "RobotDriveDevRef"=w517) -> ("error out"=w523:errorcluster, "RobotDriveDevRef"=w522:T3)  [unwired: 6 in, 1 out]
          n144 = case shown="False" w495 {
            tunnel: [-0.65 ("Output") 0.0 ("Output")] -> w496
            frame False {
            }
            frame True {
            }
          }
          n145 = call <vilib>:"WPI_RobotDriveDelayAndUpdateSafety.vi"("error in (no error)"=w523, "Delay (s)"=3.5, "RobotDriveDevRef"=w522) -> ("error out"=w515:errorcluster, "RobotDriveDevRef 2"=w516:T3)  [unwired: 7 in]
          n146 = call <vilib>:"WPI_RobotDriveTankDrive.vi"("error in (no error)"=w515, "Right axis value"=0.0, "Left axis value"=0.0, "RobotDriveDevRef"=w516) -> ("error out"=w512:errorcluster, "RobotDriveDevRef"=w510:T3)  [unwired: 5 in, 1 out]
          n147 = call <vilib>:"WPI_MotorControlSetOutput.vi"("error in (no error)"=w512, "Output"=w496, "MotorControlDevRef"=w492) -> ("error out"=w509:errorcluster, "MotorControlDevRef"=w491:T4)  [unwired: 6 in, 1 out]
          n148 = call <vilib>:"WPI_RobotDriveDelayAndUpdateSafety.vi"("error in (no error)"=w509, "Delay (s)"=2.0, "RobotDriveDevRef"=w510) -> ("error out"=w503:errorcluster, "RobotDriveDevRef 2"=w504:T3)  [unwired: 7 in]
          n149 = call <vilib>:"WPI_RobotDriveTankDrive.vi"("error in (no error)"=w503, "Right axis value"=0.0, "Left axis value"=0.6, "RobotDriveDevRef"=w504) -> ("error out"=w490:errorcluster, "RobotDriveDevRef"=w505:T3)  [unwired: 5 in, 1 out]
          n150 = call <vilib>:"WPI_MotorControlSetOutput.vi"("error in (no error)"=w490, "Output"=0.0, "MotorControlDevRef"=w491) -> ("error out"=w464:errorcluster)  [unwired: 6 in, 2 out]
          n151 = call <vilib>:"WPI_RobotDriveDelayAndUpdateSafety.vi"("error in (no error)"=w464, "Delay (s)"=1.2, "RobotDriveDevRef"=w505) -> ("error out"=w499:errorcluster, "RobotDriveDevRef 2"=w500:T3)  [unwired: 7 in]
          n152 = call <vilib>:"WPI_RobotDriveTankDrive.vi"("error in (no error)"=w499, "Right axis value"=0.0, "Left axis value"=0.0, "RobotDriveDevRef"=w500) -> ("error out"=w463:errorcluster, "RobotDriveDevRef"=w475:T3)  [unwired: 5 in, 1 out]
          n153 = call <vilib>:"WPI_MotorControlSetOutput.vi"("error in (no error)"=w463, "Output"=0.1, "MotorControlDevRef"=w461) -> ("error out"=w462:errorcluster, "MotorControlDevRef"=w453:T4)  [unwired: 6 in, 1 out]
          n154 = call <vilib>:"WPI_RobotDriveDelayAndUpdateSafety.vi"("error in (no error)"=w462, "Delay (s)"=0.025, "RobotDriveDevRef"=w475) -> ("error out"=w454:errorcluster, "RobotDriveDevRef 2"=w455:T3)  [unwired: 7 in]
          n155 = call <vilib>:"WPI_RobotDriveTankDrive.vi"("error in (no error)"=w454, "Right axis value"=0.0, "Left axis value"=0.0, "RobotDriveDevRef"=w455) -> ("error out"=w451:errorcluster, "RobotDriveDevRef"=w458:T3)  [unwired: 5 in, 1 out]
          n156 = call <vilib>:"WPI_MotorControlSetOutput.vi"("error in (no error)"=w451, "Output"=0.0, "MotorControlDevRef"=w453) -> ("error out"=w450:errorcluster)  [unwired: 6 in, 2 out]
          n157 = call <vilib>:"WPI_RobotDriveDelayAndUpdateSafety.vi"("error in (no error)"=w450, "Delay (s)"=0.1, "RobotDriveDevRef"=w458) -> ("error out"=w448:errorcluster, "RobotDriveDevRef 2"=w449:T3)  [unwired: 7 in]
          n158 = call <vilib>:"WPI_RobotDriveTankDrive.vi"("error in (no error)"=w448, "Right axis value"=0.0, "Left axis value"=0.0, "RobotDriveDevRef"=w449) -> ("error out"=w474:errorcluster, "RobotDriveDevRef"=w473:T3)  [unwired: 5 in, 1 out]
          n159 = call <vilib>:"WPI_MotorControlSetOutput.vi"("error in (no error)"=w474, "Output"=1.0, "MotorControlDevRef"=w498) -> ("error out"=w525:errorcluster, "MotorControlDevRef"=w482:T4)  [unwired: 6 in, 1 out]
          n160 = call <vilib>:"WPI_MotorControlSetOutput.vi"("error in (no error)"=w525, "Output"=-1.0, "MotorControlDevRef"=w497) -> ("error out"=w524:errorcluster, "MotorControlDevRef"=w481:T4)  [unwired: 6 in, 1 out]
          n161 = call <vilib>:"WPI_RobotDriveDelayAndUpdateSafety.vi"("error in (no error)"=w524, "Delay (s)"=0.5, "RobotDriveDevRef"=w473) -> ("error out"=w485:errorcluster, "RobotDriveDevRef 2"=w486:T3)  [unwired: 7 in]
          n162 = call <vilib>:"WPI_RobotDriveTankDrive.vi"("error in (no error)"=w485, "Right axis value"=-0.5, "Left axis value"=-0.5, "RobotDriveDevRef"=w486) -> ("error out"=w483:errorcluster, "RobotDriveDevRef"=w470:T3)  [unwired: 5 in, 1 out]
          n163 = call <vilib>:"WPI_MotorControlSetOutput.vi"("error in (no error)"=w483, "Output"=0.0, "MotorControlDevRef"=w482) -> ("error out"=w484:errorcluster)  [unwired: 6 in, 2 out]
          n164 = call <vilib>:"WPI_MotorControlSetOutput.vi"("error in (no error)"=w484, "Output"=0.0, "MotorControlDevRef"=w481) -> ("error out"=w469:errorcluster)  [unwired: 6 in, 2 out]
          n165 = call <vilib>:"WPI_RobotDriveDelayAndUpdateSafety.vi"("error in (no error)"=w469, "Delay (s)"=1.5, "RobotDriveDevRef"=w470) -> ("error out"=w465:errorcluster, "RobotDriveDevRef 2"=w466:T3)  [unwired: 7 in]
          n166 = call <vilib>:"WPI_RobotDriveTankDrive.vi"("error in (no error)"=w465, "Right axis value"=0.0, "Left axis value"=0.0, "RobotDriveDevRef"=w466) -> ()  [unwired: 5 in, 3 out]
        }
        frame "LRL", "RRR" {
          n167 = call <vilib>:"WPI_RobotDriveTankDrive.vi"("error in (no error)"=w532, "Right axis value"=0.82 ("Y axis value"), "Left axis value"=0.8 ("X axis value"), "RobotDriveDevRef"=w531) -> ("error out"=w538:errorcluster, "RobotDriveDevRef"=w537:T3)  [unwired: 5 in, 1 out]
          n168 = call <vilib>:"WPI_RobotDriveDelayAndUpdateSafety.vi"("error in (no error)"=w538, "Delay (s)"=1.4, "RobotDriveDevRef"=w537) -> ("error out"=w546:errorcluster, "RobotDriveDevRef 2"=w545:T3)  [unwired: 7 in]
          n169 = call-poly <vilib>:"WPI_RobotDriveArcadeDrive.vi"("error in (no error)"=w546, "Y axis value"=0.0, "RobotDriveDevRef"=w545) -> ("error out"=w540:errorcluster, "RobotDriveDevRef"=w543:T3)  [unwired: 6 in, 1 out]
          n170 = call <vilib>:"WPI_MotorControlSetOutput.vi"("error in (no error)"=w540, "Output"=0.0, "MotorControlDevRef"=w530) -> ("error out"=w541:errorcluster)  [unwired: 6 in, 2 out]
          n171 = call <vilib>:"WPI_MotorControlSetOutput.vi"("error in (no error)"=w541, "Output"=0.0, "MotorControlDevRef"=w529) -> ("error out"=w539:errorcluster)  [unwired: 6 in, 2 out]
          n172 = call <vilib>:"WPI_RobotDriveDelayAndUpdateSafety.vi"("error in (no error)"=w539, "Delay (s)"=0.5, "RobotDriveDevRef"=w543) -> ()  [unwired: 7 in, 2 out]
        }
      }
    }
  }
